vi "WebSocket Client Request.vi"(6 "Request Method":T2, 8 "error in":errorcluster, 10 "Websocket Command In":T1={"Command"="Get Config", "Data"=""}, 11 "WebSocket Connection in":refnum<k5>) -> (0 "error out":errorcluster, 2 "Websocket Command Out":T1, 3 "WebSocket Connection out":refnum<k5>)   [LabVIEW 2018]
uses:
  Data Def/WebSocket Request Method.ctl
  Data Def/Websocket Command.ctl
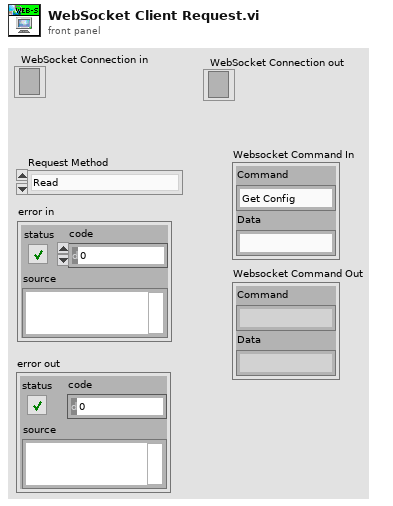
[diagram p1: front panel]
types:
  T1 = typedef "Websocket Command.ctl" = cluster{"Command":string, "Data":string}
  T2 = typedef "WebSocket Request Method.ctl" = enum16{"Read", "Write"}
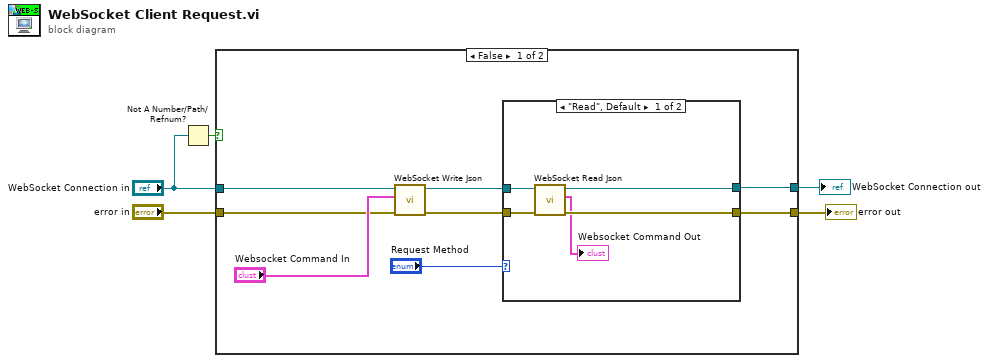
[diagram p0: block diagram]
diagram:
  n1 = Not A Number/Path/Refnum?(number/path/refnum="WebSocket Connection in") -> (NaN/Path/Refnum?=w2:bool)
  n2 = case shown="False" w2 {
    tunnel: [w9 w22] -> w5
    tunnel: [w8 w21] -> w4
    tunnel: "error in" -> [w7 w21]
    tunnel: "WebSocket Connection in" -> [w6 w22]
    frame False {
      n3 = call "WebSocket Write Json.vi"("error in"=w7, "Websocket Command"="Websocket Command In", "WebSocket Connection in"=w6) -> ("error out"=w11:errorcluster, "WebSocket Connection out"=w10:refnum<k5>)  [unwired: 7 in]
      n4 = case shown="\"Read\", Default" "Request Method" {
        tunnel: w11 -> [w18 w19]
        tunnel: w10 -> [w17 w20]
        tunnel: [w16 w19] -> w8
        tunnel: [w15 w20] -> w9
        frame "Read", Default {
          n5 = call "WebSocket Read Json.vi"("error in"=w18, "WebSocket Connection in"=w17) -> ("error out"=w16:errorcluster, "Websocket Command"=→"Websocket Command Out":T1, "WebSocket Connection out"=w15:refnum<k5>)  [unwired: 7 in]
        }
        frame "Write" {
        }
      }
    }
    frame True {
    }
  }
  "error out" <- w4
  "WebSocket Connection out" <- w5
